vi "BotSpeak_HTTP_ReadWrite.vi"() -> ()   [LabVIEW 2014]
uses:
  <userlib>/botspeak/VIs/Direct/BotSpeak_Control.ctl
  <userlib>/botspeak/VIs/SubVIs/BotSpeak_Globals.vi
panel:
  out "connection ID out":refnum<k5>
  out "data out":string
  out "error out":errorcluster
  in  "Bot Settings in":T1
  out "Bot Settings out":T1
  in  "connection ID":refnum<k5>
  in  "error in":errorcluster
  in  "To Send":string
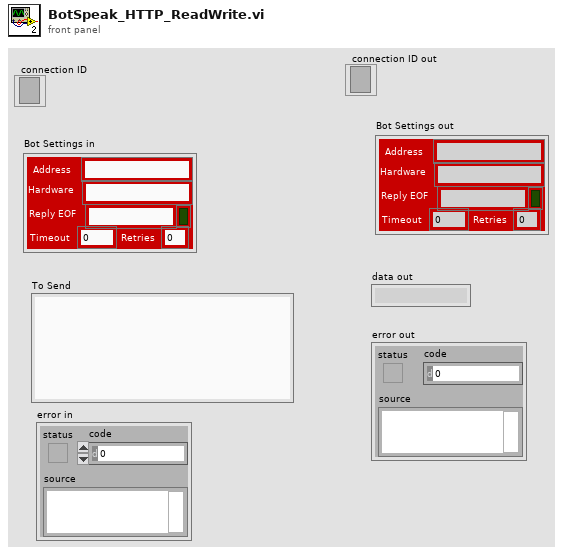
[diagram p1: front panel]
types:
  T1 = typedef "BotSpeak_Control.ctl" = cluster{"Address":string, "Reply EOF":string, "Hardware":string, "Retries":i8, "Timeout":i32, "Open?":bool}
  T2 = enum16{"Standard", "Buffered", "CRLF", "Immediate"}
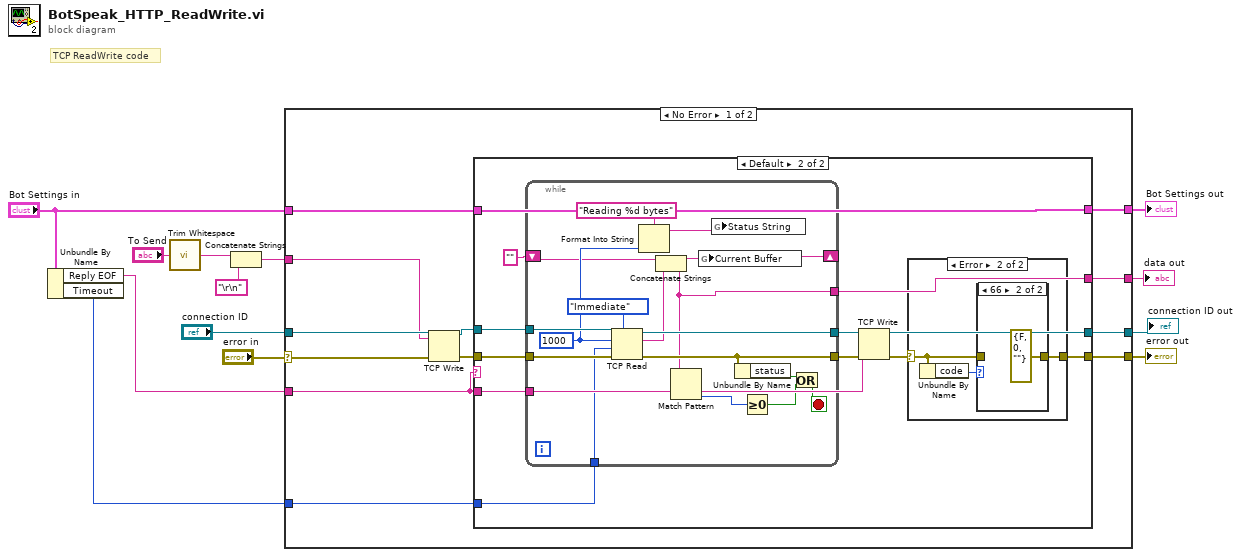
[diagram p0: block diagram]
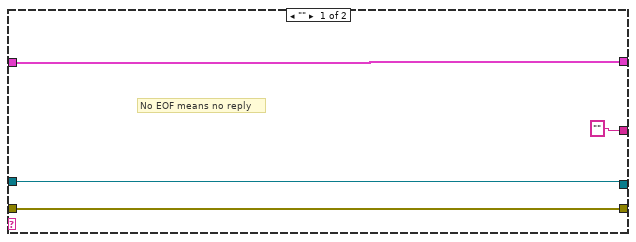
[diagram p2: hidden frame]
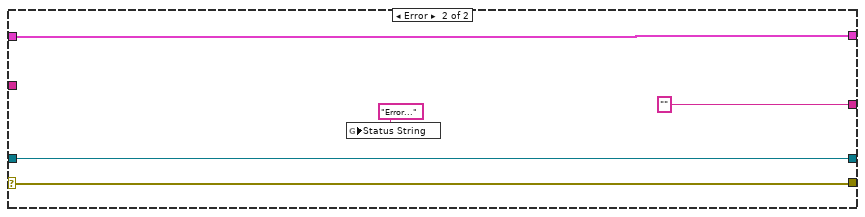
[diagram p5: hidden frame]
diagram:
  # "TCP ReadWrite code"
  n1 = Unbundle By Name("Bot Settings in") -> ("Reply EOF"=w6:string, "Timeout"=w1:i32)
  n2 = call <vilib>:"Trim Whitespace.vi"("string"="To Send") -> ("trimmed string"=w2:string)  [unwired: 1 in]
  n3 = Concatenate Strings(w2, "\r\n" ("string")) -> (w5:string)
  n4 = case shown="No Error" "error in" {
    selector: "error in" -> [w19 w67]
    tunnel: [w25 ""] -> w9
    tunnel: [w24 w67] -> w10
    tunnel: "Bot Settings in" -> [w23 w65]
    tunnel: [w22 w65] -> w11
    tunnel: "connection ID" -> [w21 w66]
    tunnel: w6 -> [w20 _]
    tunnel: w5 -> [w16 _]
    tunnel: [w15 w66] -> w4
    tunnel: w1 -> [w14 _]
    frame No Error {
      n5 = TCP Write(connection ID=w21, data in=w16, error in (no error)=w19) -> (connection ID out=w17:refnum<k5>, error out=w18:errorcluster)  [unwired: 1 in, 1 out]
      n6 = case shown="Default" w20 {
        tunnel: w20 -> [_ w34]
        tunnel: ["" w33] -> w25
        tunnel: [w28 w30] -> w24
        tunnel: w17 -> [w27 w41]
        tunnel: w18 -> [w28 w40]
        tunnel: w14 -> [_ w37]
        tunnel: w23 -> [w26 w32]
        tunnel: [w26 w32] -> w22
        tunnel: [w27 w36] -> w15
        frame "" {
          # "No EOF means no reply"
        }
        frame Default {
          n7 = while {
            tunnel: w41 -> [w64]
            tunnel: w40 -> [w63]
            tunnel: [w60] -> w39
            tunnel: [w51] -> w38
            tunnel: w37 -> [w57]
            shift-right: [w48] -> _
            shift-left: "" ("data out") -> [w56]
            tunnel: w34 -> [w54]
            tunnel: [w48] -> w33
            stop <- w49 stop-if-true
            w58 = 1000 ("bytes to read")
            n8 = TCP Read(connection ID=w64, bytes to read=w58, error in (no error)=w63, 7:T2."Immediate" ("mode (standard)"), 9:w57) -> (connection ID out=w60:refnum<k5>, data out=w55:string, error out=w51:errorcluster)
            n9 = Format Into String(format string="Reading %d bytes", w58) -> (resulting string=w61:string)  [unwired: 2 in, 1 out]
            n10 = Concatenate Strings(w56, w55) -> (w48:string)
            n11 = Match Pattern(string=w48, regular expression=w54) -> (offset past match=w53:i32)  [unwired: 1 in, 3 out]
            n12 = global write "BotSpeak_Globals.vi" "Current Buffer"(w48) -> ()
            n13 = global write "BotSpeak_Globals.vi" "Status String"(w61) -> ()
            n14 = Unbundle By Name(w51) -> ("status"=w50:bool)
            n15 = Greater Or Equal To 0?(x=w53) -> (x >= 0?=w52:bool)
            n16 = Or(x=w50, y=w52) -> (x .or. y?=w49:bool)
          }
          n17 = TCP Write(connection ID=w39, data in=w34, error in (no error)=w38) -> (connection ID out=w36:refnum<k5>, error out=w31:errorcluster)  [unwired: 1 in, 1 out]
          n18 = case shown="Error" w31 {
            selector: w31 -> [w42 w43]
            tunnel: [w42 w44] -> w30
            frame No Error {
            }
            frame Error {
              n19 = Unbundle By Name(w43) -> ("code"=w45:i32)
              n20 = case shown="66" w45 {
                tunnel: [w46 errorcluster {"status"=FALSE, "code"=0, "source"=""} ("error IO")] -> w44
                tunnel: w43 -> [w46 _]
                frame Default {
                }
                frame 66 {
                }
              }
            }
          }
        }
      }
    }
    frame Error {
      n21 = global write "BotSpeak_Globals.vi" "Status String"("Error..." ("Status String")) -> ()
    }
  }
  "Bot Settings out" <- w11
  "error out" <- w10
  "data out" <- w9
  "connection ID out" <- w4
